vi "2P power status.vi"(7 "Actions":T1=enum."Clear", 8 "Error In":errorcluster, 10 "attenuator angle in":dbl format="%#_13g", 11 "requested 2P power in":dbl format="%#_13g") -> (0 "Error Out":errorcluster, 2 "attenuator angle out":dbl, 3 "requested 2P power out":dbl)   [LabVIEW 2018]
uses:
  Controls/FGV Actions.ctl
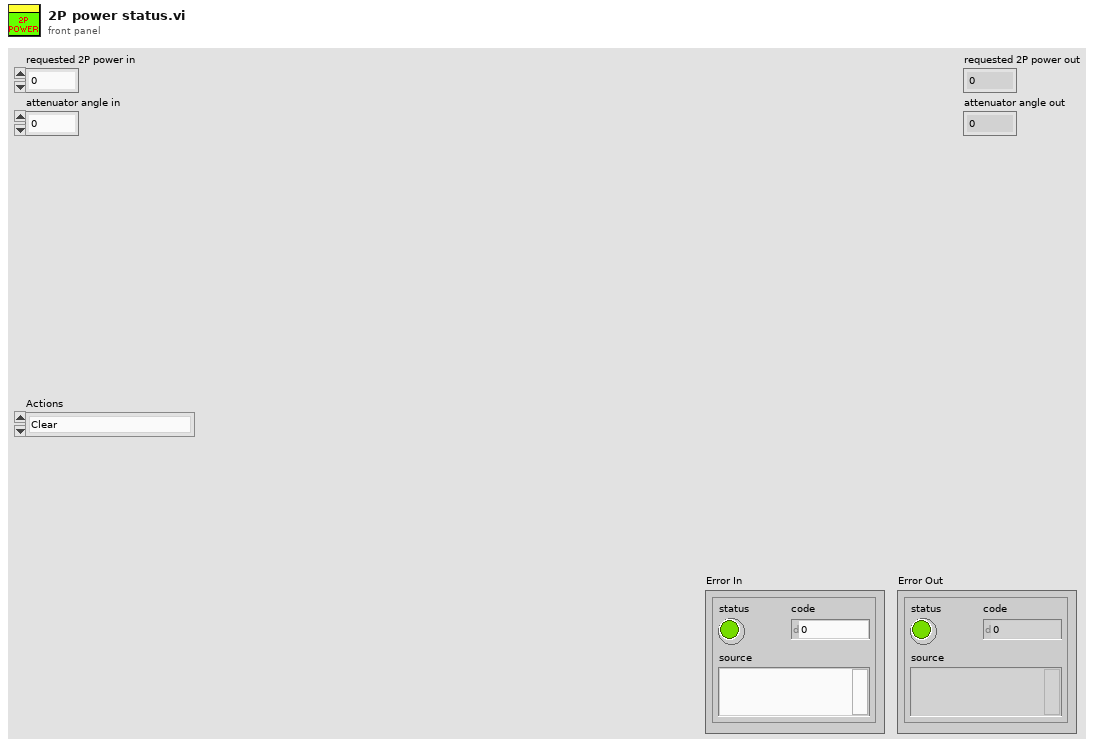
[diagram p1: front panel]
types:
  T1 = typedef "FGV Actions.ctl" = enum16{"Init", "Set", "Get", "Clear"}
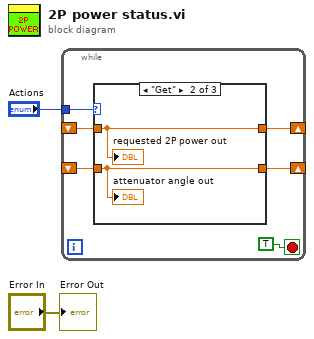
[diagram p0: block diagram]
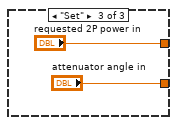
[diagram p3: hidden frame]
diagram:
  n1 = while {
    tunnel: "Actions" -> [w8]
    shift-right: [w6] -> _
    shift-left: _ -> [w4]
    shift-right: [w5] -> _
    shift-left: _ -> [w3]
    stop <- TRUE stop-if-true
    n2 = case shown="\"Get\"" w8 {
      tunnel: [_ w10 "requested 2P power in"] -> w6
      tunnel: [_ w9 "attenuator angle in"] -> w5
      tunnel: w4 -> [_ w10 _]
      tunnel: w3 -> [_ w9 _]
      frame "Init", Default {
      }
      frame "Get" {
        "requested 2P power out" <- w10
        "attenuator angle out" <- w9
      }
      frame "Set" {
      }
    }
  }
  "Error Out" <- "Error In"
